vi "AlternatorExample.vi"(10 "Boolean in 1":bool) -> (2 "Boolean out 1":bool)   [LabVIEW 2012]
panel:
  in  "Boolean in 2":bool
  out "Boolean out 2":bool
  in  "stop":bool
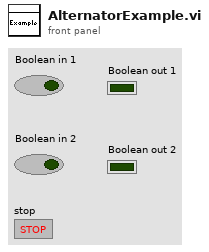
[diagram p1: front panel]
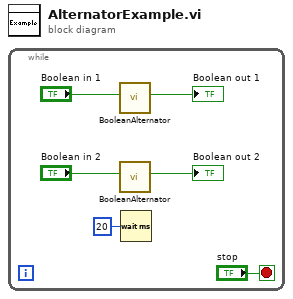
[diagram p0: block diagram]
diagram:
  n1 = while {
    stop <- "stop" stop-if-true
    n2 = call "BooleanAlternator.vi"("Boolean in"="Boolean in 1") -> ("Boolean out"=→"Boolean out 1":bool)  [unwired: 10 in]
    n3 = call "BooleanAlternator.vi"("Boolean in"="Boolean in 2") -> ("Boolean out"=→"Boolean out 2":bool)  [unwired: 10 in]
    n4 = Wait (ms)(milliseconds to wait=u32 20) -> ()  [unwired: 1 out]
  }
